vi "ModifyClassAttribute.vi"(1 "Lock time (ms)":u32, 2 "timeout in ms (-1)":i32=-1, 3 "Only unlock data? (F)":bool, 4 "Unlock data if error? (T)":bool=TRUE, 5 "error in (no error)":errorcluster) -> (17 "timeout":bool, 18 "created new":bool, 19 "error out":errorcluster)   [LabVIEW 2020, in "G#BaseClass2.lvclass"]
uses:
  G#BaseClass2.lvclass
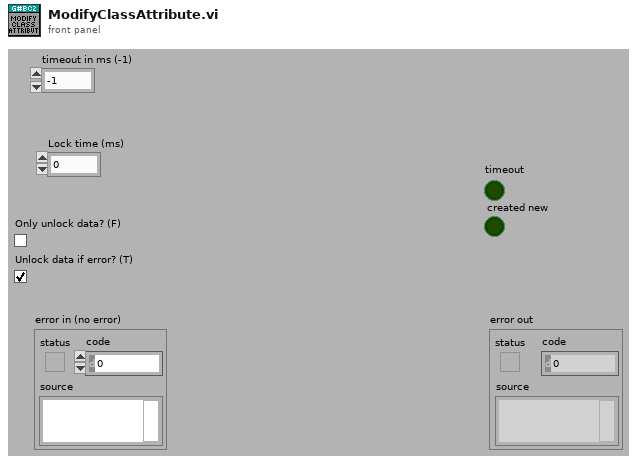
[diagram p1: front panel]
types:
  T1 = typedef "G#BaseClass2.lvclass/ClassAttributes.ctl" = cluster{"ClassAttr":i32}
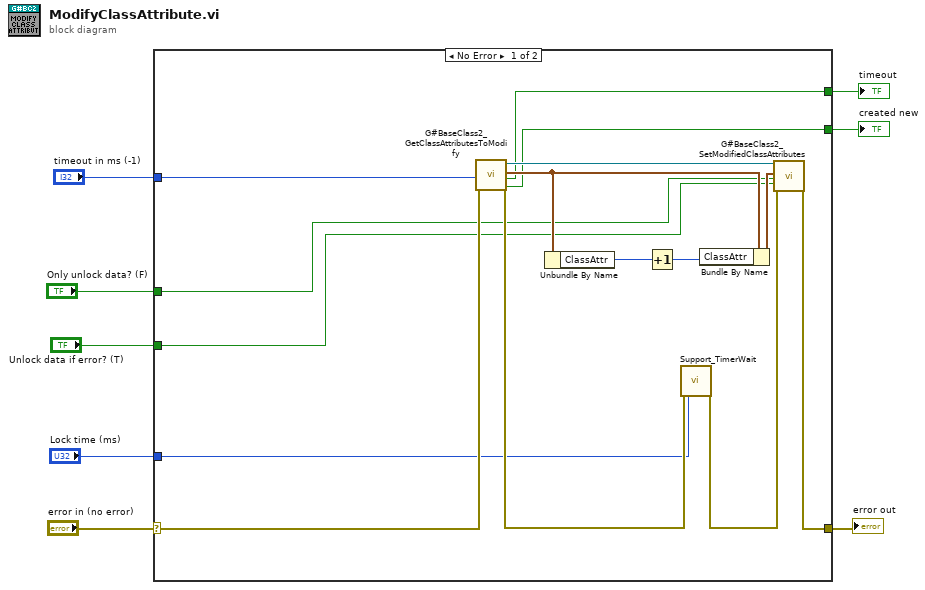
[diagram p0: block diagram]
diagram:
  n1 = case shown="No Error" "error in (no error)" {
    selector: "error in (no error)" -> [w20 w24]
    tunnel: [w21 w24] -> w7
    tunnel: "Lock time (ms)" -> [w17 _]
    tunnel: "Only unlock data? (F)" -> [w13 _]
    tunnel: "Unlock data if error? (T)" -> [w12 _]
    tunnel: "timeout in ms (-1)" -> [w11 _]
    tunnel: [w10 _] -> w2
    tunnel: [w9 _] -> w1
    frame No Error {
      n2 = call "G#BaseClass2_GetClassAttributesToModify.vi"("timeout in ms (-1)"=w11, "error in (no error)"=w20) -> ("reference out"=w22:refnum<class "G#BaseClass2.lvclass">, "class attributes"=w16:T1, "timeout"=w10:bool, "created new"=w9:bool, "error out"=w19:errorcluster)  [unwired: 12 in, 1 out]
      n3 = Unbundle By Name(w16) -> ("ClassAttr"=w15:i32)
      n4 = Increment(x=w15) -> (x+1=w14:i32)
      n5 = call "Support_TimerWait.vi"("error in (no error)"=w19, "milliseconds to wait"=w17) -> ("error out"=w18:errorcluster)  [unwired: 17 in]
      n6 = Bundle By Name(cluster=w16, "ClassAttr"=w14) -> (w23:T1)
      n7 = call "G#BaseClass2_SetModifiedClassAttributes.vi"("reference in"=w22, "attributes"=w23, "Only unlock data? (F)"=w13, "Unlock data if error? (T)"=w12, "error in (no error)"=w18) -> ("error out"=w21:errorcluster)  [unwired: 13 in, 1 out]
    }
    frame Error {
    }
  }
  "error out" <- w7
  "timeout" <- w2
  "created new" <- w1
